vi "Average_curves.vi"(9 "Array in":dbl[](array[numeric]), 10 "Counter":i8, 11 "file path (dialog if empty)":path) -> (1 "Array out":dbl[](array[numeric]), 2 "Resampled i(B) array":dbl[][](array[numeric]), 3 "Mean I(B)":dbl[](array[numeric]))   [LabVIEW 2015]
uses:
  <vilib>/Analysis/baseanly.llb/Mean (DBL).vi
  <vilib>/Utility/file.llb/Read Delimited Spreadsheet (DBL).vi
  <vilib>/Analysis/NI_AALBase.lvlib
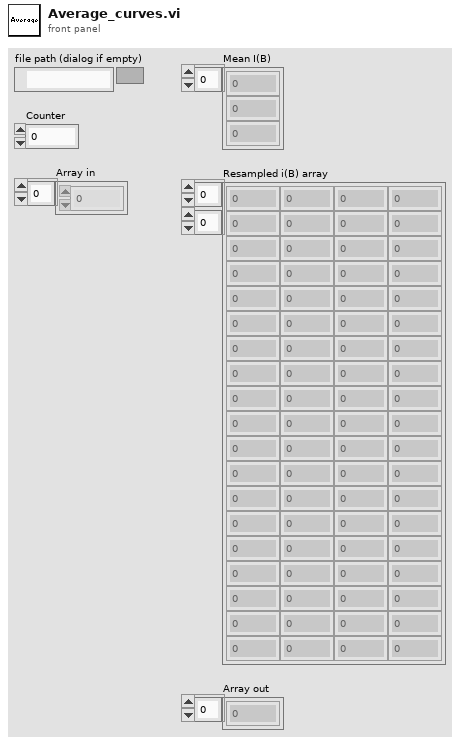
[diagram p1: front panel]
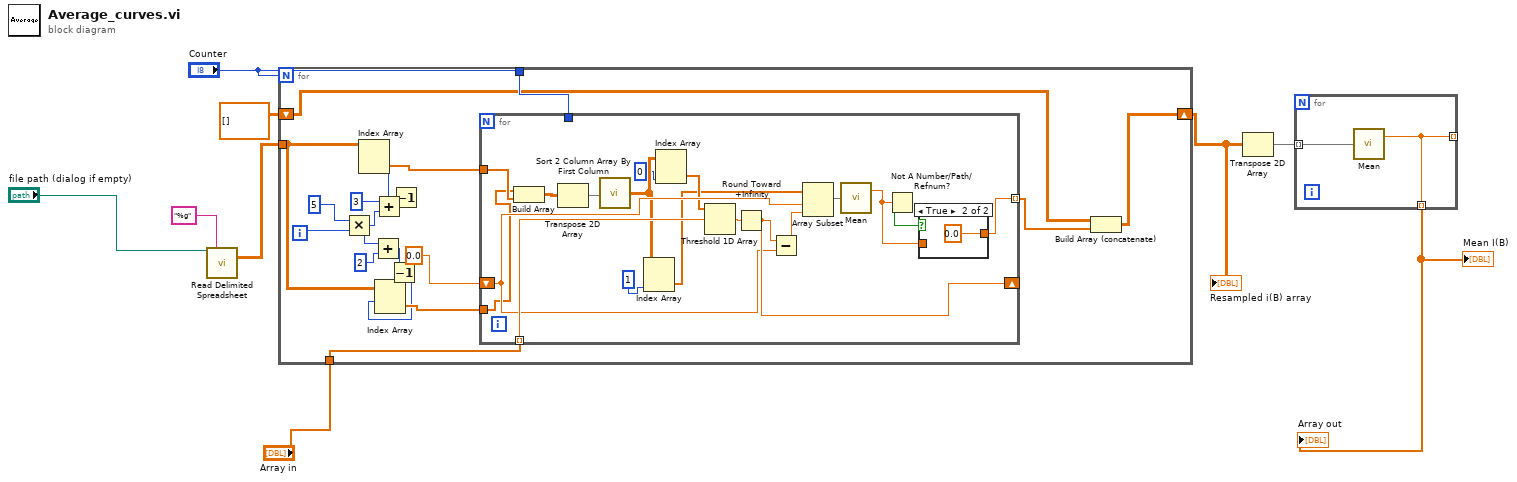
[diagram p0: block diagram]
diagram:
  n1 = call-poly <vilib>:"Read Delimited Spreadsheet.vi"("file path (dialog if empty)"="file path (dialog if empty)", "format (%.3f)"="%g") -> ("all rows"=w3:dbl[][])  [unwired: 8 in, 5 out]
  n2 = for {
    N: "Counter" -> [_]
    tunnel: w3 -> [w19]
    tunnel: "Array in" -> [w23]
    tunnel: "Counter" -> [w16]
    shift-right: [w11] -> w5
    shift-left: dbl[][] [] -> [w10]
    i -> [w15]
    n3 = Multiply(x=5, y=w15) -> (x*y=w22:i32)
    n4 = Add(x=w22, y=2 ("x")) -> (x+y=w20:i32)
    n5 = Add(x=3, y=w22) -> (x+y=w25:i32)
    n6 = Decrement(x=w20) -> (x-1=w14:i32)
    n7 = Index Array(array=w19, index (row)=w14) -> (element=w18:dbl[])  [unwired: 1 in]
    n8 = Decrement(x=w25) -> (x-1=w13:i32)
    n9 = Index Array(array=w19, index (row)=w13) -> (element=w24:dbl[])  [unwired: 1 in]
    n10 = for {
      tunnel: w24 -> [w36]
      tunnel: w23 -> [w42] mode=indexing
      tunnel: w18 -> [w28]
      shift-right: [w41] -> _
      shift-left: 0.0 -> [w39]
      tunnel: w16 -> [_]
      tunnel: [w37] -> w12 mode=indexing
      n11 = Build Array(w28, w36) -> (w35:dbl[][])
      n12 = Transpose 2D Array(2D array=w35) -> (transposed array=w34:dbl[][])
      n13 = call "Sort 2 Column Array By First Column.vi"("2D array to sort"=w34) -> ("Sorted array"=w33:dbl[][])
      n14 = Index Array(array=w33, index (col)=1 ("index (row)")) -> (element=w29:dbl[])  [unwired: 1 in]
      n15 = Index Array(array=w33, index (col)=0 ("index (row)")) -> (element=w32:dbl[])  [unwired: 1 in]
      n16 = Threshold 1D Array(2:w42, 3:w32) -> (0:w44:dbl)  [unwired: 1 in]
      n17 = Round Toward +Infinity(x=w44) -> (ceil(x): smallest int >= x=w41:dbl)
      n18 = Subtract(x=w41, y=w39) -> (x-y=w43:dbl)
      n19 = Array Subset(array=w29, index=w39, length=w43) -> (w40:dbl[])
      n20 = call-poly <vilib>:"Mean.vi"("X"=w40) -> ("mean"=w38:dbl)  [unwired: 1 out]
      n21 = Not A Number/Path/Refnum?(number/path/refnum=w38) -> (NaN/Path/Refnum?=w45:bool)
      n22 = case shown="True" w45 {
        tunnel: [w46 0.0] -> w37
        tunnel: w38 -> [w46 _]
        frame False {
        }
        frame True {
        }
      }
    }
    n23 = Build Array (concatenate)(w10, w12) -> (w11:dbl[][])
  }
  "Resampled i(B) array" <- w5
  n24 = Transpose 2D Array(2D array=w5) -> (transposed array=w9:dbl[][])
  n25 = for {
    tunnel: [w48] -> _ mode=indexing
    tunnel: w9 -> [w49] mode=indexing
    tunnel: [w48] -> w7 mode=indexing
    n26 = call-poly <vilib>:"Mean.vi"("X"=w49) -> ("mean"=w48:dbl)  [unwired: 1 out]
  }
  "Mean I(B)" <- w7
  "Array out" <- w7
